vi "move.vi"(8 "error in (no error)":errorcluster, 11 "Human in":refnum<class "Human.lvclass">) -> (0 "error out":errorcluster, 2 "message":string, 3 "Human out":refnum<class "Human.lvclass">)   [LabVIEW 2017, in "Human.lvclass"]
uses:
  Human.lvclass
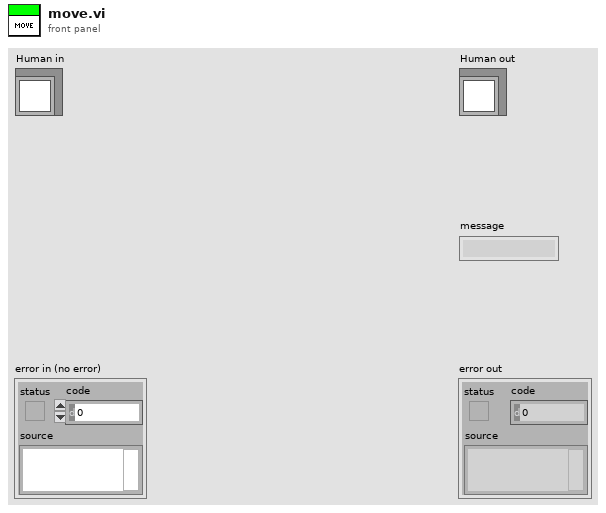
[diagram p1: front panel]
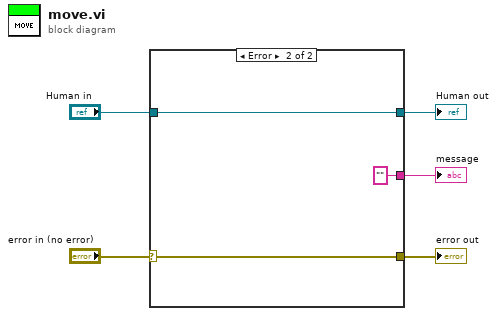
[diagram p0: block diagram]
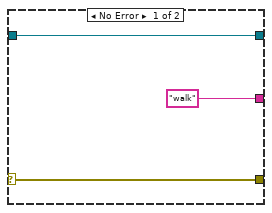
[diagram p2: hidden frame]
diagram:
  n1 = case shown="Error" "error in (no error)" {
    selector: "error in (no error)" -> [w8 w9]
    tunnel: [w8 w9] -> w4
    tunnel: "Human in" -> [w7 w11]
    tunnel: [w7 w11] -> w2
    tunnel: ["walk" ""] -> w1
    frame No Error {
    }
    frame Error {
    }
  }
  "error out" <- w4
  "Human out" <- w2
  "message" <- w1
